vi "pf Get Camera Property F.vi"(8 "error in (no error)":errorcluster, 10 "pProperty":string, 11 "iPort":i32) -> (0 "error out":errorcluster, 3 "function return":sgl)   [LabVIEW 2025, in "Photonfocus_Toolkit.lvlib"]
doc: "PFCONFIG_API float pfGetCameraPropertyF(const char* pProperty);"
uses:
  Photonfocus_Toolkit.lvlib
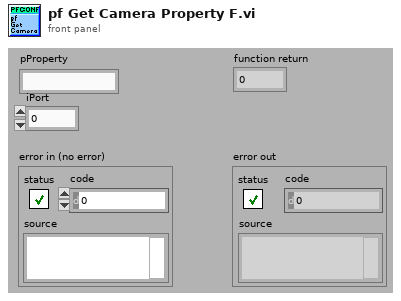
[diagram p1: front panel]
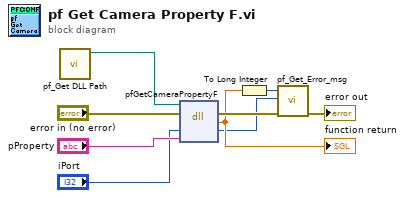
[diagram p0: block diagram]
diagram:
  n1 = call "pf_Get DLL Path.vi"() -> ("DLL path"=w7:path)  [unwired: 1 in, 10 out]
  n2 = dll-call lib="S:/Progetti/Photonfocus/Codice/DEV/PFConfig_lvlib/PFConfig.*" fn="pfGetCameraPropertyF"(path in=w7, error in="error in (no error)", "iPort"="iPort", "pProperty"="pProperty") -> (error out=w6:errorcluster, "return type"=w4:sgl, "iPort"=w1:i32)  [unwired: 2 in, 1 out]
  "function return" <- w4
  n3 = To Long Integer(number=w4) -> (32bit integer=w3:i32)
  n4 = call "pf_Get_Error_msg.vi"("error in (no error)"=w6, "iPort"=w1, "error code"=w3) -> ("error out"=→"error out":errorcluster)  [unwired: 8 out]
